vi "motor XY setMeng.vi"(6 "Motor settings Z":cluster{"Vmax (mm/s)":sgl, "Acc (mm/s/s)":sgl}, 8 "Motor serial numbers":i32[](array[numeric]), 9 "Motor settings (X,Y)":cluster{"Vmax (mm/s)":sgl, "Acc (mm/s/s)":sgl}, 10 "Array":errorcluster[](array[cluster]), 11 "Array 2":refnum<k7>[](array[refnum])) -> (1 "Array 3":errorcluster[](array[cluster]), 3 "Array 4":refnum<k7>[](array[refnum]))   [LabVIEW 2014]
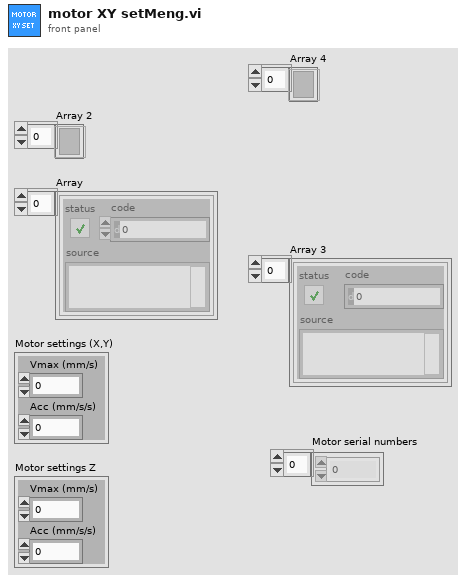
[diagram p1: front panel]
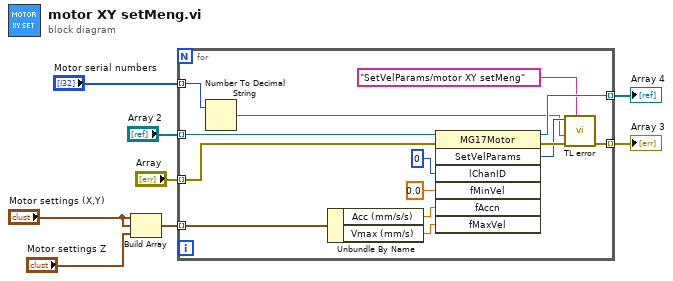
[diagram p0: block diagram]
diagram:
  n1 = Build Array("Motor settings (X,Y)", "Motor settings (X,Y)", "Motor settings Z") -> (w3:cluster{"Vmax (mm/s)":sgl, "Acc (mm/s/s)":sgl}[])
  n2 = for {
    tunnel: "Array 2" -> [w21] mode=indexing
    tunnel: "Array" -> [w22] mode=indexing
    tunnel: [w18] -> w2 mode=indexing
    tunnel: [w13] -> w4 mode=indexing
    tunnel: w3 -> [w17] mode=indexing
    tunnel: "Motor serial numbers" -> [w11] mode=indexing
    n3 = Number To Decimal String(number=w11) -> (decimal integer string=w10:string)  [unwired: 1 in]
    n4 = Unbundle By Name(w17) -> ("Acc (mm/s/s)"=w16:sgl, "Vmax (mm/s)"=w15:sgl)
    n5 = invoke class="MG17Motor" method="SetVelParams"(reference=w21, error in=w22, "lChanID"=0, "fMinVel"=sgl 0.0, "fAccn"=w16, "fMaxVel"=w15) -> (reference out=w18:refnum<k7>, error out=w14:errorcluster, "SetVelParams"=w12:i32)  [unwired: 1 in, 4 out]
    n6 = call "TL error.vi"("Input string"="SetVelParams/motor XY setMeng", "error in (no error)"=w14, "Serial number of motor"=w10, "Return Code"=w12) -> ("error out"=w13:errorcluster)  [unwired: 7 in]
  }
  "Array 3" <- w4
  "Array 4" <- w2
